vi "角度至弧度（单位）.vi"(1 "degree":dbl[unit]) -> (0 "radian":dbl[unit])   [LabVIEW 2012, in "几何工具.lvlib"]
doc: "功能：\n\n角度转换为弧度。\n\n输入：角度，单位为度。\n\n输出：弧度。\n\ncsxcs_366创建。"
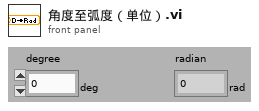
[diagram p1: front panel]
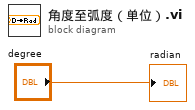
[diagram p0: block diagram]
diagram:
  "radian" <- "degree"
